vi "Initialize Test Device Modbus Client Serial.vi"(0 "PLBB in":refnum<class "Test Device.lvclass">, 1 "protocol (RTU)":enum16{"RTU", "ASCII", "TCP"}(ring), 2 "station address (1)":u8=1, 3 "timeout, ms (300)":u32=300, 5 "port":refnum<visa-resource-name>, 7 "baud rate (115200)":u32=115200, 9 "data bits (8)":u16=8, 11 "error in (no error)":errorcluster, 12 "parity (even)":enum16{"None", "Odd", "Even", "Mark", "Space"}(ring)=enum."Even", 13 "stop bits (1.0)":u16(ring)=10 items=["1.0"=10, "1.5"=15, "2.0"=20], 14 "flow control (none)":u16(ring) items=["None", "XON/XOFF", "RTS/CTS", "XON/XOFF & RTS/CTS", "DTR/DSR", "XON/XOFF & DTR/DSR"]) -> (4 "PLBB out":refnum<class "Test Device.lvclass">, 15 "error out":errorcluster)   [LabVIEW 2015, in "Test Device.lvclass"]
uses:
  Test Device.lvclass
  <vilib>/plasmapper/PL BlackBox Modbus CLient/PL BlackBox Modbus Client.lvclass
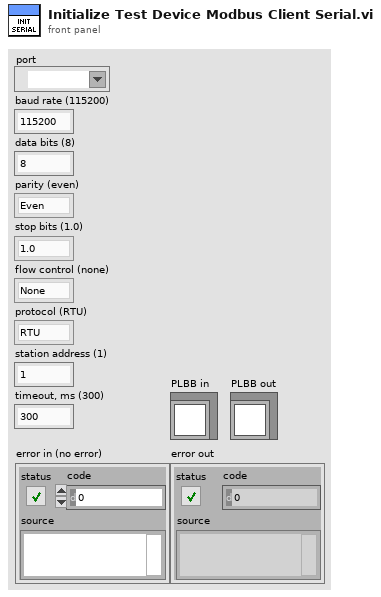
[diagram p1: front panel]
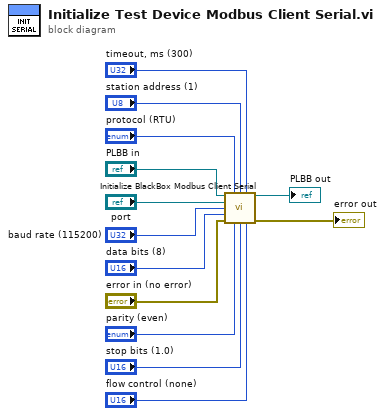
[diagram p0: block diagram]
diagram:
  n1 = call <vilib>:"Initialize BlackBox Modbus Client Serial.vi"("PLBB in"="PLBB in", "protocol (RTU)"="protocol (RTU)", "station address (1)"="station address (1)", "timeout, ms (300)"="timeout, ms (300)", "port"="port", "baud rate (115200)"="baud rate (115200)", "data bits (8)"="data bits (8)", "error in (no error)"="error in (no error)", "parity (even)"="parity (even)", "stop bits (1.0)"="stop bits (1.0)", "flow control (none)"="flow control (none)") -> ("PLBB out"=→"PLBB out":refnum<class "Test Device.lvclass">, "error out"=→"error out":errorcluster)  [unwired: 3 in]
